vi "cross_correlate.vi"(6 "invert channels":bool[](array[boolean])=[FALSE, FALSE], 7 "fly-back?":bool, 8 "pixel finished?":bool, 10 "maximum bit depth":i8, 11 "integration cluster in":T1={"channel 0"=0, "channel 1"=0, "fly-back heap address"=0, "fly-forward heap address"=0, "xc buffer"=[0, 0, 0, 0, 0]}) -> (3 "integration cluster out":T1)   [LabVIEW 2010]
uses:
  integration_cluster.ctl
  <vilib>/rvi/DataTransferAndStorage/Container/XNode/niFpgaContainer.xnode
  <vilib>/rvi/Memory/Memory_Emulation/nirvimemoryEmulationManagerCache_GetValue.vi
  <vilib>/rvi/DataTransferAndStorage/Container/Common/niFpgaContainerGetUniqueNameForEmu.vi
  <vilib>/rvi/Memory/Memory_Emulation/nirvimemoryEmulationManagerCache_InsertValue.vi
  <vilib>/Utility/error.llb/Clear Errors.vi
  <vilib>/rvi/Memory/Memory_Emulation/nirvimemoryEmulationManagerCache_SetValue.vi
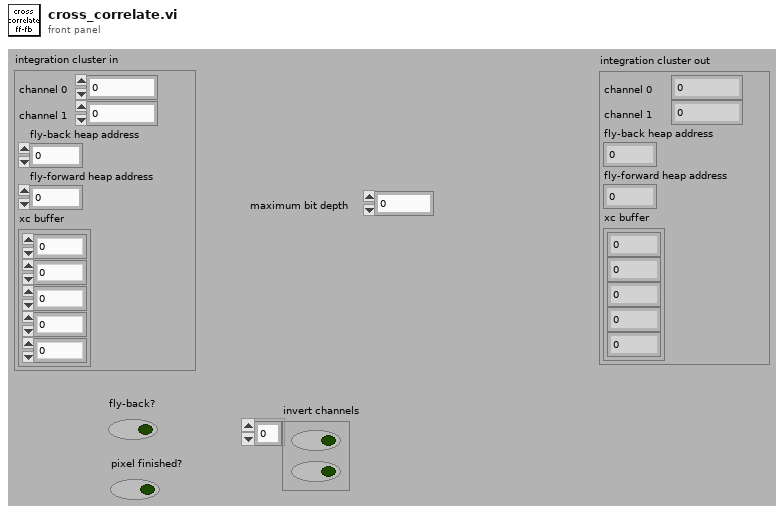
[diagram p1: front panel]
types:
  T1 = typedef "integration_cluster.ctl" = cluster{"channel 0":u32, "channel 1":u32, "fly-back heap address":u32, "fly-forward heap address":u32, "xc buffer":u32[]}
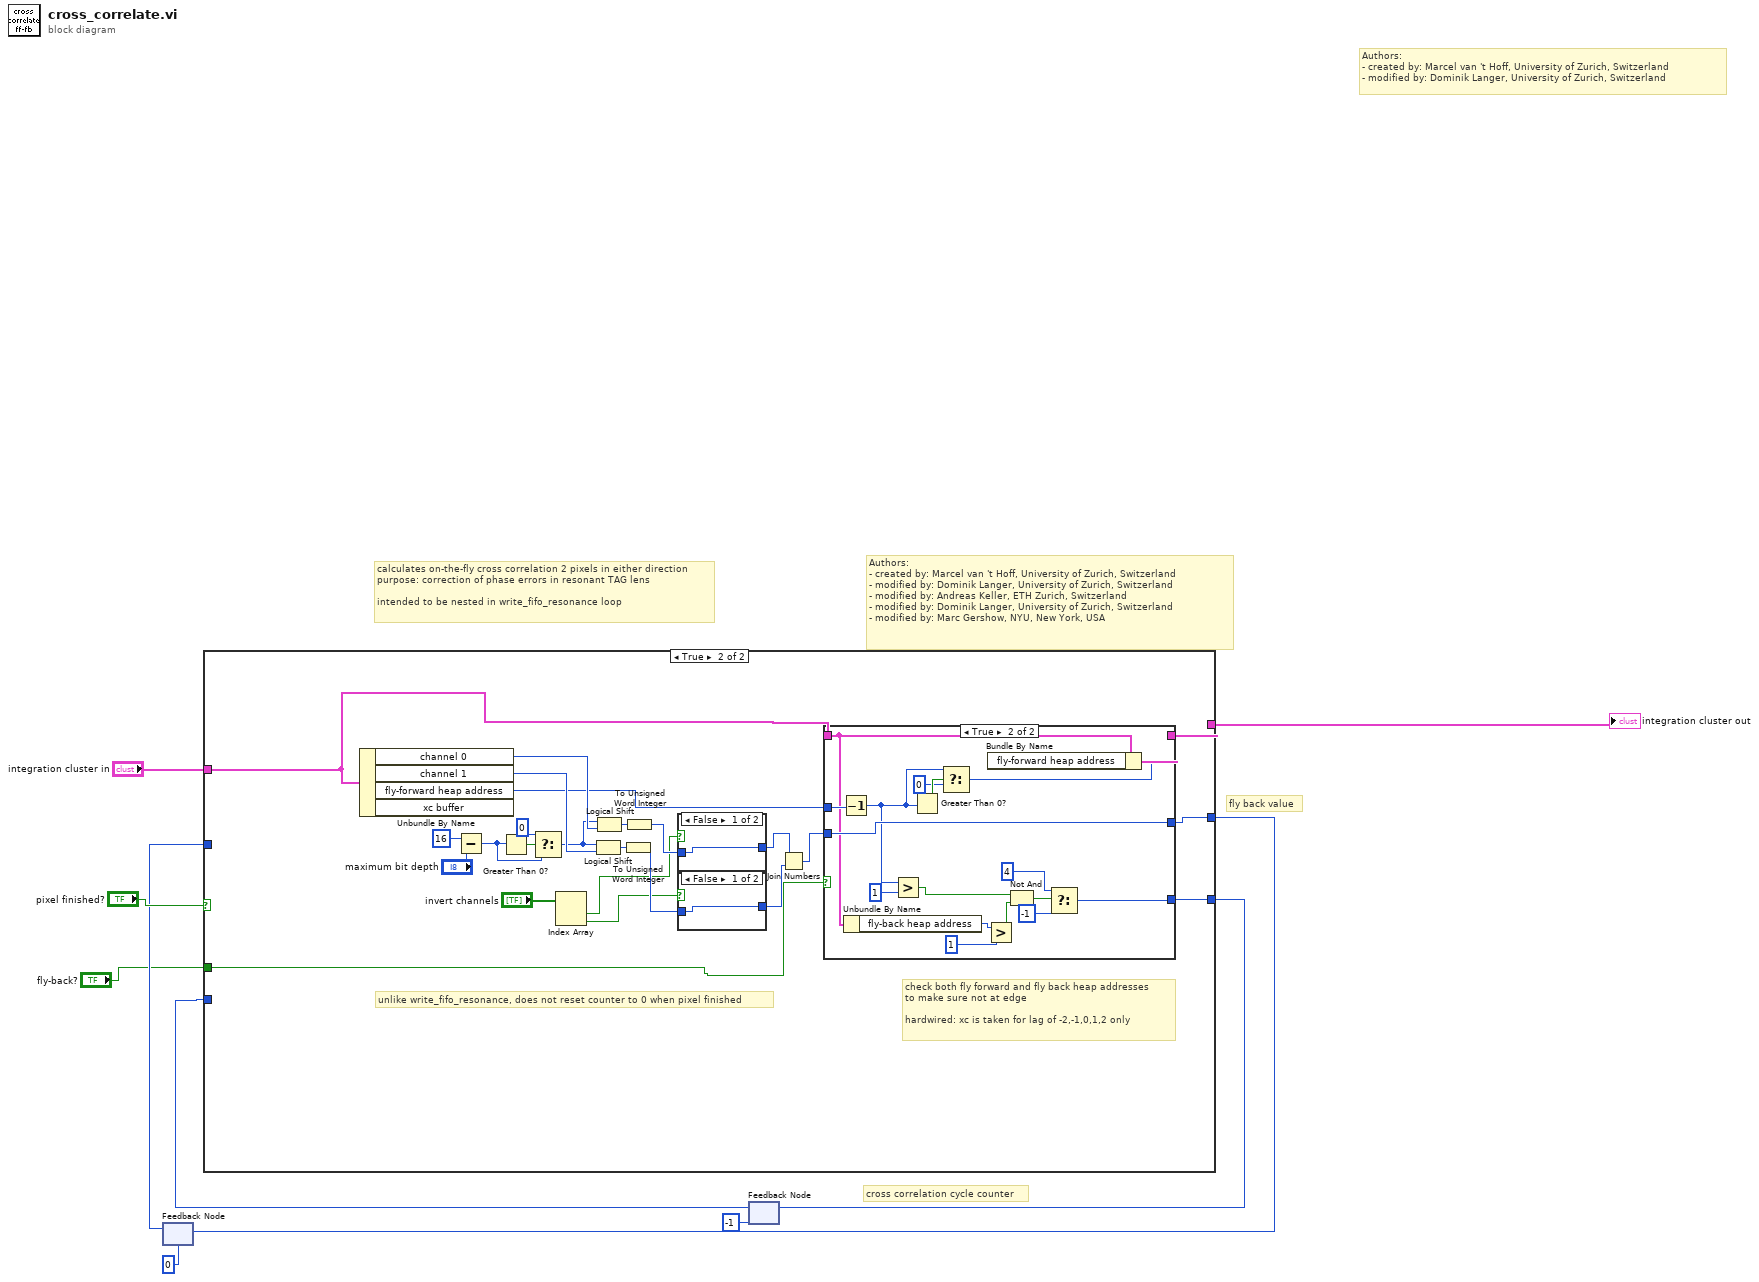
[diagram p0: block diagram]
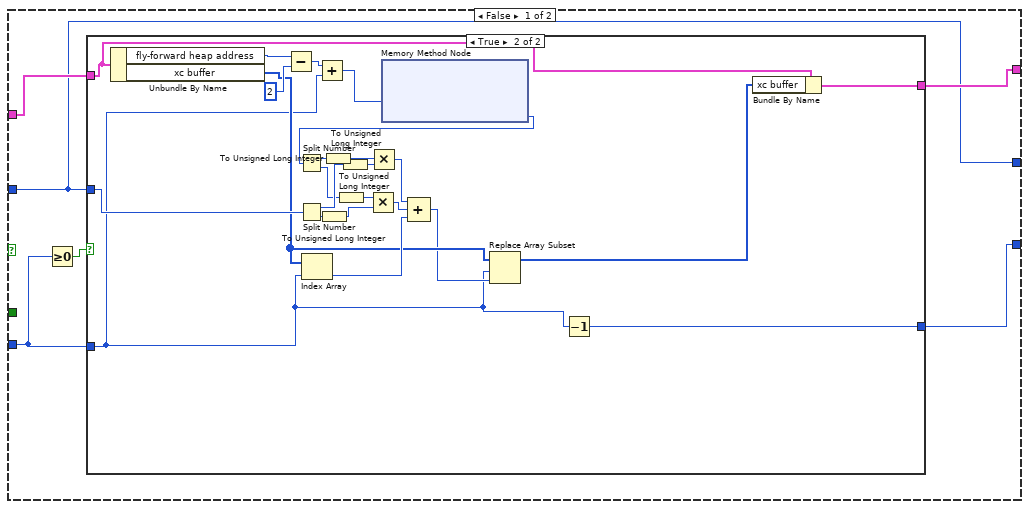
[diagram p2: hidden frame]
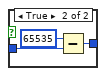
[diagram p4: hidden frame]
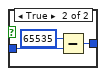
[diagram p5: hidden frame]
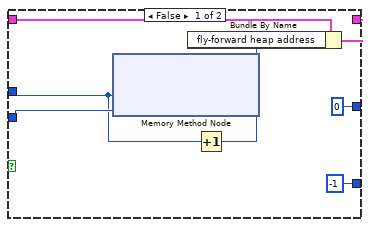
[diagram p6: hidden frame]
diagram:
  # "cross correlation cycle counter"
  # "fly back value"
  # "calculates on-the-fly cross correlation 2 pixels in either direction\npurpose: correction of phase errors in resonant TAG lens\n\nintended to be nested in write_fifo_resonance loop"
  # "Authors: \n- created by: Marcel van 't Hoff, University of Zurich, Switzerland\n- modified by: Dominik Langer, University of Zurich, Switzerland\n- modified by: Andreas Keller, ETH Zurich, Switzerland\n- modified by: Dominik Langer, University of Zurich, Switzerland\n- modified by: Marc Gershow, NYU, New York, USA"
  # "Authors: \n- created by: Marcel van 't Hoff, University of Zurich, Switzerland\n- modified by: Dominik Langer, University of Zurich, Switzerland"
  n1 = feedback #1(u32 0) -> (w6:u32)
  n2 = feedback #2(i16 -1 ("f")) -> (w2:i16)
  n3 = case shown="True" "pixel finished?" {
    tunnel: "integration cluster in" -> [w16 w176]
    tunnel: [w13 w175] -> w8
    tunnel: [w11 w171] -> w7
    tunnel: w6 -> [w11 _]
    tunnel: "fly-back?" -> [_ w170]
    tunnel: [w12 w169] -> w3
    tunnel: w2 -> [w15 _]
    frame False {
      n4 = Greater Or Equal To 0?(x=w15) -> (x >= 0?=w14:bool)
      n5 = case shown="True" w14 {
        tunnel: w16 -> [w18 w23]
        tunnel: w15 -> [w17 w20]
        tunnel: w11 -> [_ w39]
        tunnel: [w18 w21] -> w13
        tunnel: [w17 w19] -> w12
        frame False {
        }
        frame True {
          n6 = Unbundle By Name(w23) -> ("fly-forward heap address"=w42:u32, "xc buffer"=w25:u32[])
          n7 = Subtract(x=w42, y=u32 2) -> (x-y=w40:u32)
          n8 = Split Number(x=w39) -> (hi(x)=w35:u16, lo(x)=w33:u16)
          n9 = Index Array(array=w25, index=w20) -> (element=w30:u32)
          n10 = Add(x=w40, y=w20) -> (x+y=w38:u32)
          n11 = To Unsigned Long Integer(number=w33) -> (unsigned 32bit integer=w26:u32)
          n12 = To Unsigned Long Integer(number=w35) -> (unsigned 32bit integer=w28:u32)
          n13 = xnode ("Memory Method Node")("Address"=w38) -> ("Data"=w37:u32)  [unwired: 1 in, 1 out]
          n14 = Split Number(x=w37) -> (hi(x)=w36:u16, lo(x)=w34:u16)
          n15 = To Unsigned Long Integer(number=w36) -> (unsigned 32bit integer=w29:u32)
          n16 = To Unsigned Long Integer(number=w34) -> (unsigned 32bit integer=w27:u32)
          n17 = Multiply(x=w27, y=w26) -> (x*y=w31:u32)
          n18 = Multiply(x=w29, y=w28) -> (x*y=w32:u32)
          n19 = Compound Arithmetic op=ADD(w32, w31, w30) -> (w24:u32)
          n20 = Replace Array Subset(array=w25, new element=w24, index=w20) -> (w22:u32[])
          n21 = Decrement(x=w20) -> (x-1=w19:i16)
          n22 = Bundle By Name(cluster=w23, "xc buffer"=w22) -> (w21:T1)
        }
      }
    }
    frame True {
      # "check both fly forward and fly back heap addresses\nto make sure not at edge \n\nhardwired: xc is taken for lag of -2,-1,0,1,2 only"
      # "unlike write_fifo_resonance, does not reset counter to 0 when pixel finished"
      n23 = Unbundle By Name(w176) -> ("channel 0"=w186:u32, "channel 1"=w187:u32, "fly-forward heap address"=w182:u32)  [unwired: 1 out]
      n24 = Subtract(x=i8 16, y="maximum bit depth") -> (x-y=w189:i8)
      n25 = Greater Than 0?(x=w189) -> (x > 0?=w188:bool)
      n26 = Select(t=i8 0 ("f"), s=w188, f=w189) -> (s? t:f=w185:i8)
      n27 = Index Array(array="invert channels") -> (element #1=w178:bool, element #2=w177:bool)  [unwired: 2 in]
      n28 = Logical Shift(y=w185, x=w187) -> (x << y=w184:u32)
      n29 = Logical Shift(y=w185, x=w186) -> (x << y=w183:u32)
      n30 = To Unsigned Word Integer(number=w184) -> (unsigned 16bit integer=w180:u16)
      n31 = To Unsigned Word Integer(number=w183) -> (unsigned 16bit integer=w181:u16)
      n32 = case shown="False" w178 {
        tunnel: [w197 w199] -> w174
        tunnel: w181 -> [w197 w198]
        frame False {
        }
        frame True {
          n33 = Subtract(x=u16 65535, y=w198) -> (x-y=w199:u16)
        }
      }
      n34 = case shown="False" w177 {
        tunnel: [w193 w195] -> w173
        tunnel: w180 -> [w193 w194]
        frame False {
        }
        frame True {
          n35 = Subtract(x=u16 65535, y=w194) -> (x-y=w195:u16)
        }
      }
      n36 = Join Numbers(hi=w174, lo=w173) -> ((hi.lo)=w172:u32)
      n37 = case shown="True" w170 {
        tunnel: w182 -> [w204 w347]
        tunnel: w176 -> [w207 w341]
        tunnel: [w206 w349] -> w175
        tunnel: w172 -> [w205 w344]
        tunnel: [u32 0 w344] -> w171
        tunnel: [i16 -1 ("f") w333] -> w169
        frame False {
          n38 = xnode ("Memory Method Node")("Address"=w204, "Data"=w205) -> ()  [unwired: 1 in, 1 out]
          n39 = Increment(x=w204) -> (x+1=w203:u32)
          n40 = Bundle By Name(cluster=w207, "fly-forward heap address"=w203) -> (w206:T1)
        }
        frame True {
          n41 = Decrement(x=w347) -> (x-1=w343:u32)
          n42 = Unbundle By Name(w341) -> ("fly-back heap address"=w340:u32)
          n43 = Greater?(x=w343, y=u32 1) -> (0:w338:bool)
          n44 = Greater Than 0?(x=w343) -> (x > 0?=w346:bool)
          n45 = Select(t=w343, s=w346, f=u32 0) -> (s? t:f=w348:u32)
          n46 = Greater?(x=w340, y=u32 1) -> (0:w337:bool)
          n47 = Bundle By Name(cluster=w341, "fly-forward heap address"=w348) -> (w349:T1)
          n48 = Not And(1:w337, 2:w338) -> (0:w336:bool)
          n49 = Select(t=i16 4 ("f"), s=w336, f=i16 -1) -> (s? t:f=w333:i16)
        }
      }
    }
  }
  "integration cluster out" <- w8
  n50 = feedback-in #1(w7) -> ()
  n51 = feedback-in #2(w3) -> ()
